vi "Read moveDestination.vi"(8 "error in (no error)":errorcluster, 11 "KST101 in":refnum<class "KST101.lvclass">) -> (0 "error out":errorcluster, 2 "moveDestination":dbl, 3 "KST101 out":refnum<class "KST101.lvclass">)   [LabVIEW 2016, in "Stepper Motor Controller.lvlib" / "KST101.lvclass"]
uses:
  KST101.lvclass
  KST101.lvclass/KST101.ctl
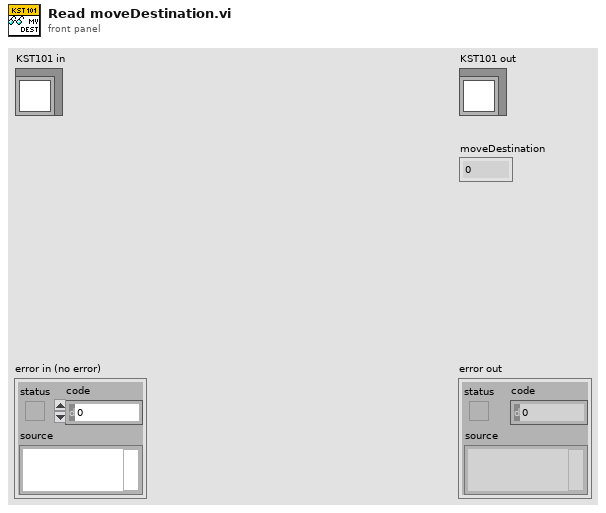
[diagram p1: front panel]
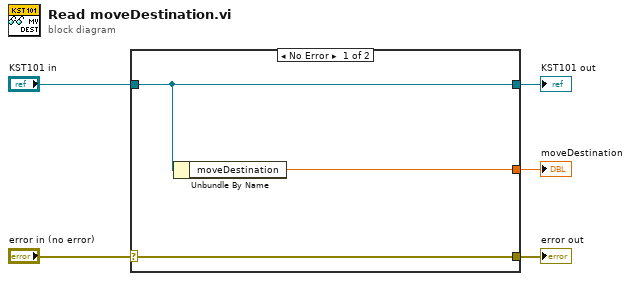
[diagram p0: block diagram]
diagram:
  n1 = case shown="No Error" "error in (no error)" {
    selector: "error in (no error)" -> [w8 w9]
    tunnel: [w8 w9] -> w4
    tunnel: [w7 w10] -> w2
    tunnel: "KST101 in" -> [w7 w10]
    tunnel: [w6 _] -> w1
    frame No Error {
      n2 = Unbundle By Name(w7) -> ("moveDestination"=w6:dbl)
    }
    frame Error {
    }
  }
  "error out" <- w4
  "KST101 out" <- w2
  "moveDestination" <- w1
